vi "CRC-32-IEEE 802.3.vi"(5 "Frame in":u8[](array[numeric]) format="%x") -> (1 "CRC32[]":u8[](array[numeric]) format="%.0x", 2 "CRC32Value":u32 format="%x")   [LabVIEW 2018]
panel:
  in  "CRC Buffer":u32=4294967295 format="%x"
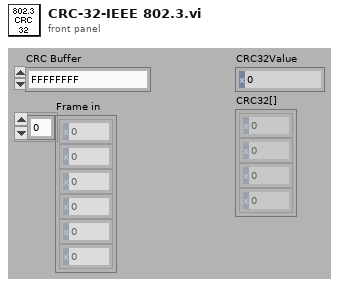
[diagram p1: front panel]
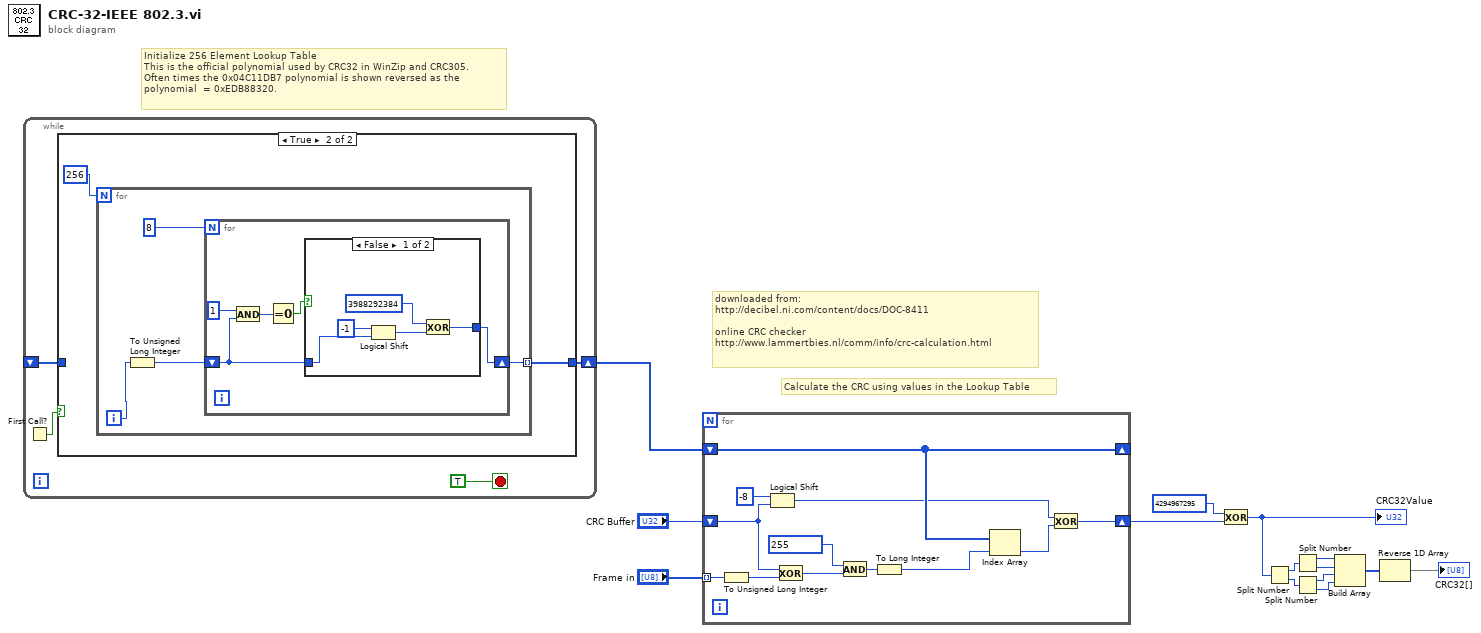
[diagram p0: block diagram]
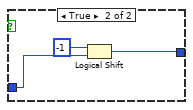
[diagram p3: hidden frame]
diagram:
  # "downloaded from: \nhttp://decibel.ni.com/content/docs/DOC-8411\n\nonline CRC checker\nhttp://www.lammertbies.nl/comm/info/crc-calculation.html"
  # "Calculate the CRC using values in the Lookup Table"
  # "Initialize 256 Element Lookup Table\nThis is the official polynomial used by CRC32 in WinZip and CRC305.\nOften times the 0x04C11DB7 polynomial is shown reversed as the\npolynomial  = 0xEDB88320."
  n1 = while {
    shift-right: [w16] -> w13
    shift-left: _ -> [w15]
    stop <- TRUE stop-if-true
    n2 = First Call?() -> (First Call?: T/F=w17:bool)
    n3 = case shown="True" w17 {
      tunnel: [w19 w20] -> w16
      tunnel: w15 -> [w19 _]
      frame False {
      }
      frame True {
        n4 = for {
          N: 256 -> [_]
          tunnel: [w22] -> w20 mode=indexing
          i -> [w24]
          n5 = To Unsigned Long Integer(number=w24) -> (unsigned 32bit integer=w23:u32)
          n6 = for {
            N: 8 -> [_]
            shift-right: [w26] -> w22
            shift-left: w23 -> [w30]
            n7 = And(x=u32 1, y=w30) -> (x .and. y?=w28:u32)
            n8 = Equal To 0?(x=w28) -> (x = 0?=w27:bool)
            n9 = case shown="False" w27 {
              tunnel: w30 -> [w35 w38]
              tunnel: [w31 w36] -> w26
              frame False {
                n10 = Logical Shift(y=-1, x=w35) -> (x << y=w33:u32)
                n11 = Exclusive Or(1:w33, 2:u32 3988292384 ("x")) -> (0:w31:u32)
              }
              frame True {
                n12 = Logical Shift(y=-1, x=w38) -> (x << y=w36:u32)
              }
            }
          }
        }
      }
    }
  }
  n13 = for {
    tunnel: "Frame in" -> [w45] mode=indexing
    shift-right: [w40] -> w12
    shift-left: "CRC Buffer" -> [w46]
    shift-right: [w50] -> _
    shift-left: w13 -> [w50]
    n14 = To Unsigned Long Integer(number=w45) -> (unsigned 32bit integer=w44:u32)
    n15 = Logical Shift(y=-8, x=w46) -> (x << y=w39:u32)
    n16 = Exclusive Or(1:w44, 2:w46) -> (0:w47:u32)
    n17 = And(x=u32 255, y=w47) -> (x .and. y?=w43:u32)
    n18 = To Long Integer(number=w43) -> (32bit integer=w42:i32)
    n19 = Index Array(array=w50, index=w42) -> (element=w41:u32)
    n20 = Exclusive Or(1:w41, 2:w39) -> (0:w40:u32)
  }
  n21 = Exclusive Or(1:w12, 2:u32 4294967295 ("x")) -> (0:w9:u32)
  "CRC32Value" <- w9
  n22 = Split Number(x=w9) -> (hi(x)=w8:u16, lo(x)=w7:u16)
  n23 = Split Number(x=w8) -> (hi(x)=w6:u8, lo(x)=w5:u8)
  n24 = Split Number(x=w7) -> (hi(x)=w4:u8, lo(x)=w3:u8)
  n25 = Build Array(w6, w5, w4, w3) -> (w2:u8[])
  n26 = Reverse 1D Array(array=w2) -> (reversed array=→"CRC32[]":u8[])
